vi "convert total to active channel indices.vi"(10 "channelConfig":T1[](array[typedef]), 11 "AbsoluteChannelIndices":u16[](array[numeric])) -> (0 "error out":errorcluster, 2 "activeChannelIndices":u16[](array[numeric]))   [LabVIEW 2018]
uses:
  type defs/channelControl.ctl
  RT/Type Defs/channelScalingTypes.ctl
  RT/Type Defs/scalingMethods.ctl
  <vilib>/Utility/error.llb/Error Cluster From Error Code.vi
  <vilib>/ErrorRing/Error Ring.xnode
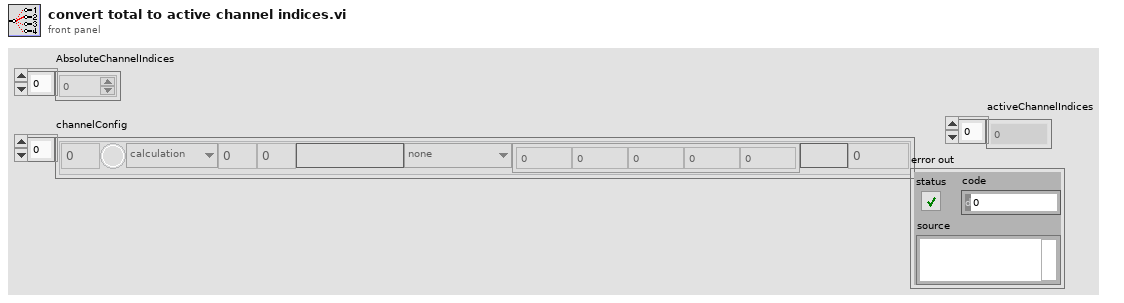
[diagram p1: front panel]
types:
  T1 = typedef "channelControl.ctl" = cluster{"index":u16, "active":bool, "channelType":T2, "module":u16, "terminal":u16, "channelName":string, "scalingMethod":T3, "scalingParameters":dbl[], "scaledUnits":string, "tempOffset":dbl}
  T2 = typedef "channelScalingTypes.ctl" = enum16{"calculation", "measurement", "scanivalve", "output", "digital"}
  T3 = typedef "scalingMethods.ctl" = enum16{"none", "linear", "thermocouple", "polynomial", "encoder", "RTD"}
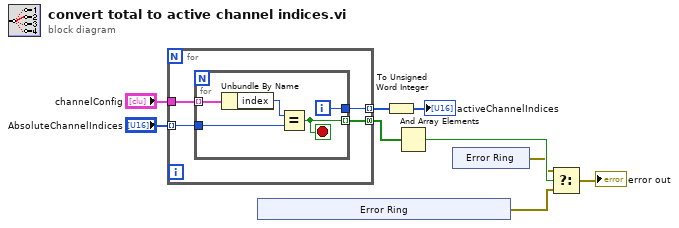
[diagram p0: block diagram]
diagram:
  n1 = for {
    tunnel: "channelConfig" -> [w13]
    tunnel: "AbsoluteChannelIndices" -> [w12] mode=indexing
    tunnel: [w11] -> w5 mode=concatenating
    tunnel: [w10] -> w7 mode=indexing
    n2 = for {
      tunnel: w13 -> [w18] mode=indexing
      tunnel: w12 -> [w16]
      tunnel: [w15] -> w11 mode=indexing
      tunnel: [w14] -> w10
      i -> [w14]
      stop <- w15 stop-if-true
      n3 = Unbundle By Name(w18) -> ("index"=w17:u16)
      n4 = Equal?(x=w17, y=w16) -> (x = y?=w15:bool)
    }
  }
  n5 = xnode "Error Ring"() -> ("error out"=w2:errorcluster)
  n6 = To Unsigned Word Integer(number=w7) -> (unsigned 16bit integer=→"activeChannelIndices":u16[])
  n7 = And Array Elements(Boolean array=w5) -> (logical AND=w4:bool)
  n8 = xnode "Error Ring"() -> ("error out"=w3:errorcluster)
  n9 = Select(t=w3, s=w4, f=w2) -> (s? t:f=→"error out":errorcluster)
